vi "RGseriesSeria210216CeramicPS1.vi"() -> ()   [LabVIEW 2015]
uses:
  <vilib>/Instr/_visa.llb/VISA Configure Serial Port (Instr).vi
  <userlib>/caLab/Private/Get_PV-1D.vi
  <userlib>/caLab/Private/Put_DBL-1D_PV-1D.vi
panel:
  out "read Current":string
  out "read Voltage":string
  out "concatenated string":string
  out "ReadWait":i16
  out "WriteWait":i16
  in  "APX:PS2_T_RV":dbl
  out "APX:PS2_V_EV":dbl format="%.3f"
  out "APX:PS2_I_EV":dbl format="%.3f"
  out "Ilim_factor":dbl
  out "Vlim_factor":dbl
  out "SSE:Tsample":dbl
  in  "I lower limit":dbl
  in  "V lower limit":dbl
  in  "I upper limit":dbl=2.8
  in  "V upper limit":dbl=18.0
  out "APX:PS2_Ct":dbl
  out "APX:PS2_Rzero":dbl
  in  "Heater":u16(ring) items=["Ceramic W/Mo", "Kanthal A-1"]
  out "APX:Theater":dbl
  out "APX:PS2_R_MV":dbl format="%.2f"
  in  "REMOTE/LOCAL":bool
  out "PS2_P_MV":dbl format="%.2f"
  in  "APX:PS2_I_RV":dbl min=0.0 max=0.5 step=0.002
  in  "APX:PS2_OUT":bool
  in  "stop":bool
  out "APX:PS2_I_MV":dbl format="%.3g"
  out "APX:PS2_V_MV":dbl format="%.3g"
  in  "VISA resource name":refnum<visa-resource-name>="COM12"
  in  "APX:PS2_V_RV":dbl min=0.0 max=8.0 step=0.05
  # "COM20"
  # "#2"
  # "Sample Heater Control"
  # "COM12"
  # "V"
  # "A"
  # "Max 1.2A/0.4x0.1wire"
  # "W"
  # "ohm"
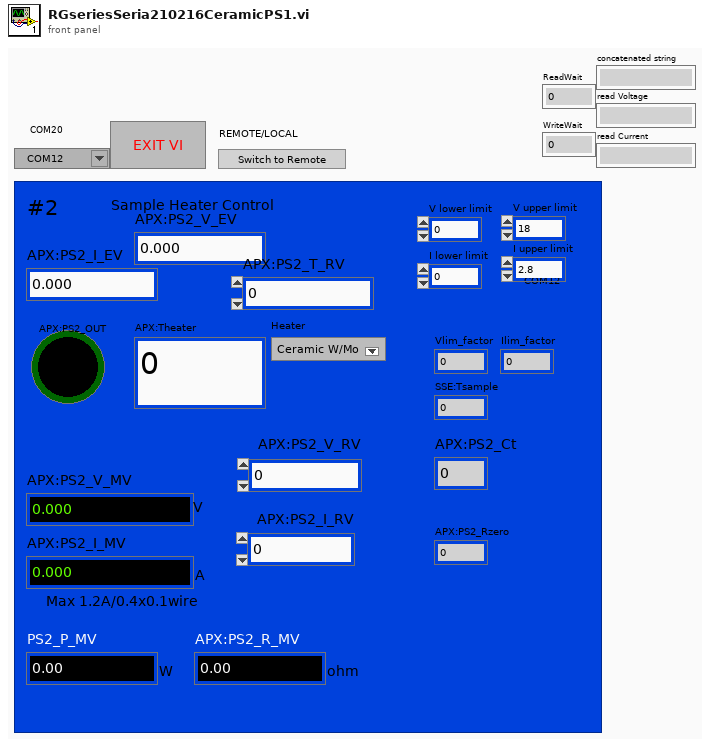
[diagram p1: front panel]
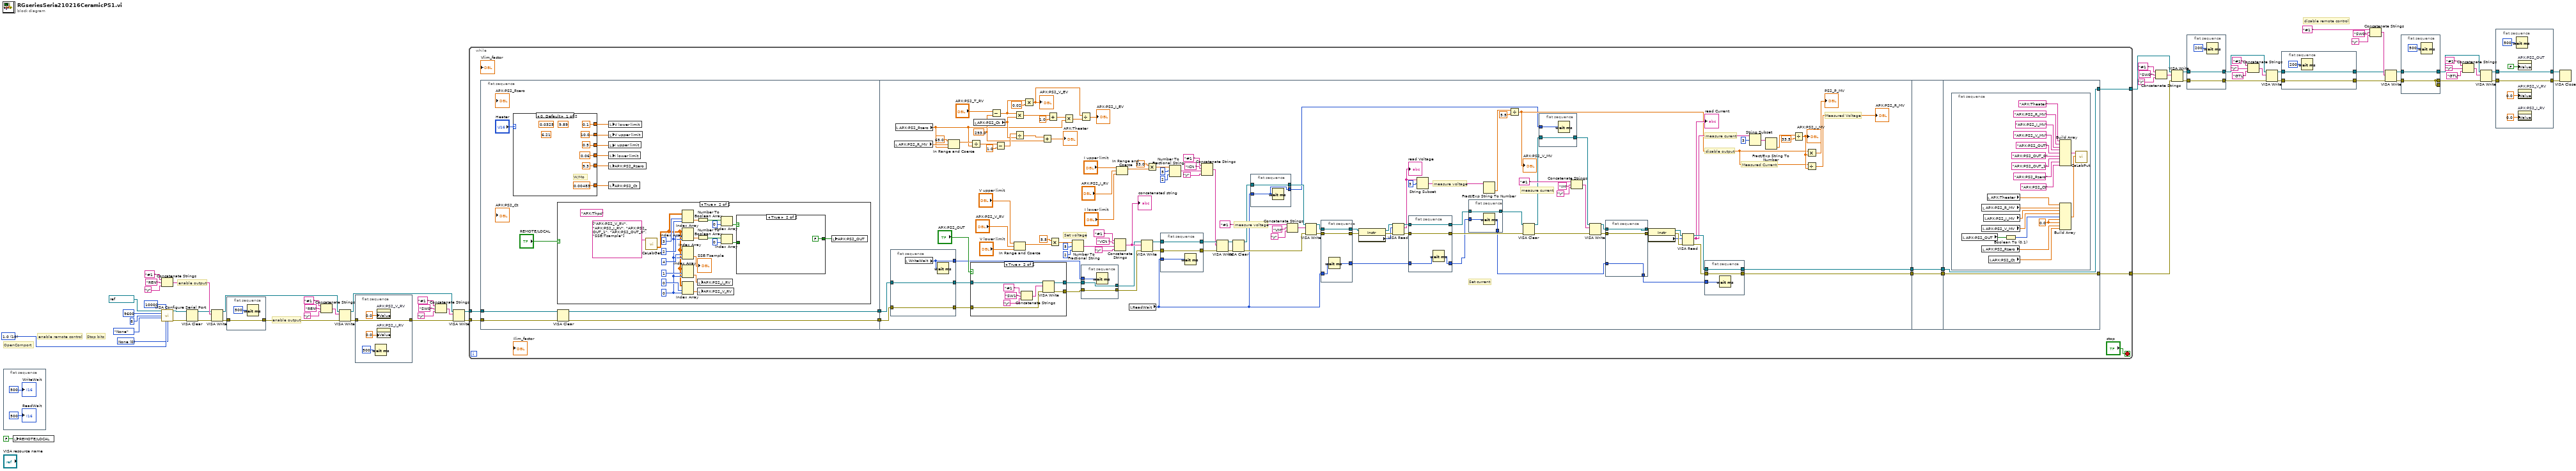
[diagram p0: block diagram]
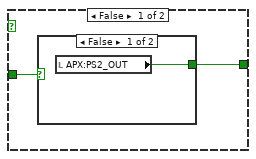
[diagram p3: hidden frame]
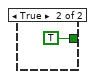
[diagram p4: hidden frame]
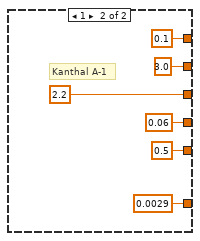
[diagram p5: hidden frame]
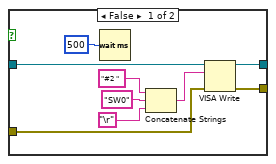
[diagram p6: hidden frame]
diagram:
  w54 = u16 0 items=["None", "XON/XOFF", "RTS/CTS", "XON/XOFF & RTS/CTS", "DTR/DSR", "XON/XOFF & DTR/DSR"] ("flow control (0:none)")
  w55 = u16 10 items=["1.0"=10, "1.5"=15, "2.0"=20] ("stop bits (10: 1 bit)")
  # "enable output"
  # "disable remote control"
  # "OpenComport"
  # "Stop bits"
  # "enable remote control"
  # "enable output"
  n1 = flat-sequence {
    frame #0 {
      "WriteWait" <- i16 500 ("WriteWait")
      "ReadWait" <- i16 500 ("ReadWait")
    }
  }
  n2 = local write "REMOTE/LOCAL"(FALSE ("REMOTE/LOCAL")) -> ()
  n3 = Concatenate Strings("#1 " ("initial string"), "REN" ("string"), "\r") -> (w53:string)
  n4 = call-poly "VISA Configure Serial Port"("VISA resource name"=refnum<visa-resource-name> "COM20", "timeout (10sec)"=u32 10000, "baud rate (9600)"=u32 9600, "data bits (8)"=u16 8, "parity (0:none)"=enum16{"None", "Odd", "Even", "Mark", "Space"}."None", "stop bits (10: 1 bit)"=w55, "flow control (0:none)"=w54) -> ("VISA resource name out"=w4:refnum<visa-resource-name>, "error out"=w3:errorcluster)  [unwired: 7 in]
  n5 = VISA Clear(VISA resource name=w4, error in (no error)=w3) -> (VISA resource name out=w1:refnum<visa-resource-name>, error out=w2:errorcluster)
  n6 = VISA Write(VISA resource name=w1, write buffer=w53, error in (no error)=w2) -> (VISA resource name out=w27:refnum<visa-resource-name>, error out=w20:errorcluster)  [unwired: 1 out]
  n7 = flat-sequence {
    tunnel: w20 -> [w70]
    tunnel: [w70] -> w21
    frame #0 {
      n8 = Wait (ms)(milliseconds to wait=u32 500) -> ()  [unwired: 1 out]
    }
  }
  n9 = Concatenate Strings("#1 " ("initial string"), "REN" ("string"), "\r") -> (w22:string)
  n10 = VISA Write(VISA resource name=w27, write buffer=w22, error in (no error)=w21) -> (VISA resource name out=w26:refnum<visa-resource-name>, error out=w19:errorcluster)  [unwired: 1 out]
  n11 = flat-sequence {
    tunnel: [w74] -> w40
    tunnel: w19 -> [w74]
    frame #0 {
      n12 = Wait (ms)(milliseconds to wait=u32 500) -> ()  [unwired: 1 out]
      n13 = property on="APX:PS2_V_RV" class="DigNum (strict)"("Value"=0.0 ("VCN_REQ")) -> ()  [unwired: 2 in, 2 out]
      n14 = property on="APX:PS2_I_RV" class="DigNum (strict)"("Value"=0.0 ("APX:RG183_I_RV")) -> ()  [unwired: 2 in, 2 out]
    }
  }
  n15 = Concatenate Strings("#1 " ("format string"), "SW0" ("initial string"), "\r" ("input 1")) -> (w52:string)
  n16 = VISA Write(VISA resource name=w26, write buffer=w52, error in (no error)=w40) -> (VISA resource name out=w42:refnum<visa-resource-name>, error out=w41:errorcluster)  [unwired: 1 out]
  n17 = while {
    tunnel: w42 -> [w84]
    tunnel: w41 -> [w85]
    tunnel: [w81] -> w39
    tunnel: [w80] -> w38
    stop <- "stop" stop-if-true
    n18 = flat-sequence {
      tunnel: w84 -> [w89]
      tunnel: w85 -> [w87]
      tunnel: [w86] -> w78
      tunnel: [w88] -> w77
      tunnel: [w198] -> w83
      tunnel: [w197] -> w82
      tunnel: w78 -> [w158]
      tunnel: w77 -> [w159]
      tunnel: w83 -> [w302]
      tunnel: w82 -> [w301]
      tunnel: [w301] -> w76
      tunnel: [w302] -> w75
      tunnel: [w304] -> w80
      tunnel: [w303] -> w81
      tunnel: w76 -> [w304]
      tunnel: w75 -> [w303]
      frame #0 {
        n19 = case shown="0, Default" "Heater" {
          tunnel: [0.00483 ("APX:PS2_Ct") 0.0029 ("APX:PS2_Ct")] -> w94
          tunnel: [9.3 ("APX:PS2_Rzero") 0.5 ("APX:PS2_Rzero")] -> w95
          tunnel: [0.5 2.2] -> w96
          tunnel: [10.0 3.0] -> w97
          tunnel: [0.1 0.1] -> w91
          tunnel: [0.06 0.06] -> w90
          frame 0, Default {
            (unwired) 9.89 ("APX:PS2_Rzero")
            (unwired) 0.0325 ("APX:PS2_Ct")
            (unwired) 6.21 ("APX:PS2_Rzero")
            # "W/Mo"
          }
          frame 1 {
            # "Kanthal A-1"
          }
        }
        n20 = case shown="True" "REMOTE/LOCAL" {
          frame False {
          }
          frame True {
            w100 = 0 ("disabled index (col)")
            (unwired) "APX:Thpc"
            n21 = call-poly "CaLabGet.vi"("PV Names"=string[] ["APX:PS2_V_RV", "APX:PS2_I_RV", "APX:PS2_OUT_1", "APX:PS2_OUT_0", "SSE:Tsample"]) -> ("Value Array (number)"=w99:dbl[][])  [unwired: 8 in, 6 out]
            n22 = Index Array(array=w99, index (row)=3 ("disabled index (row)"), index (col)=w100) -> (element=w107:dbl)
            n23 = Index Array(array=w99, index (row)=2, index (col)=w100) -> (element=w113:dbl)
            n24 = Index Array(array=w99, index (row)=4, index (col)=w100) -> (element=→"SSE:Tsample":dbl)
            n25 = Index Array(array=w99, index (row)=1, index (col)=w100) -> (element=w102:dbl)
            n26 = Index Array(array=w99, index (row)=0, index (col)=w100) -> (element=w103:dbl)
            n27 = Number To Boolean Array(number=w107) -> (Boolean array=w109:bool[])
            n28 = Number To Boolean Array(number=w113) -> (Boolean array=w112:bool[])
            n29 = local write "APX:PS2_I_RV"(w102) -> ()
            n30 = local write "APX:PS2_V_RV"(w103) -> ()
            n31 = Index Array(array=w109, index=0) -> (element=w106:bool)
            n32 = Index Array(array=w112, index=0) -> (element=w105:bool)
            n33 = case shown="True" w106 {
              tunnel: w105 -> [w119 _]
              tunnel: [w118 FALSE] -> w104
              frame False {
                n34 = case shown="False" w119 {
                  tunnel: [w120 TRUE] -> w118
                  frame False {
                    n35 = local read "APX:PS2_OUT"() -> (w120:bool)
                  }
                  frame True {
                  }
                }
              }
              frame True {
              }
            }
            n36 = local write "APX:PS2_OUT"(w104) -> ()
          }
        }
        n37 = VISA Clear(VISA resource name=w89, error in (no error)=w87) -> (VISA resource name out=w88:refnum<visa-resource-name>, error out=w86:errorcluster)
        n38 = local write "V lower limit"(w91) -> ()
        n39 = local write "V upper limit"(w97) -> ()
        n40 = local write "I upper limit"(w96) -> ()
        n41 = local write "I lower limit"(w90) -> ()
        n42 = local write "APX:PS2_Rzero"(w95) -> ()
        n43 = local write "APX:PS2_Ct"(w94) -> ()
      }
      frame #1 {
        w172 = 293.0 ("y")
        # "measure current"
        # "measure voltage"
        # "measure voltage"
        # "measure curent"
        # "Measured Voltage"
        # "Measured Current"
        # "Set current"
        # "Set voltage"
        # "disable output"
        n44 = flat-sequence {
          tunnel: w159 -> [w260]
          tunnel: w158 -> [w259]
          tunnel: [w260] -> w156
          tunnel: [w259] -> w157
          tunnel: [w258] -> w155
          frame #0 {
            n45 = local read "WriteWait"() -> (w258:i16)
            n46 = Wait (ms)(milliseconds to wait=w258) -> ()  [unwired: 1 out]
          }
        }
        n47 = local read "APX:PS2_R_MV"() -> (w185:dbl)
        n48 = local read "APX:PS2_Rzero"() -> (w167:dbl)
        n49 = In Range and Coerce(upper limit=65.0, x=w185, lower limit=w167) -> (coerced(x)=w183:dbl)  [unwired: 1 out]
        n50 = Divide(x=w183, y=w167) -> (x/y=w182:dbl)
        n51 = case shown="True" "APX:PS2_OUT" {
          tunnel: w156 -> [w270 w279]
          tunnel: w157 -> [w269 w278]
          tunnel: [w268 w277] -> w196
          tunnel: [w267 w276] -> w195
          frame False {
            n52 = Wait (ms)(milliseconds to wait=u32 500) -> ()  [unwired: 1 out]
            n53 = Concatenate Strings("#2 " ("format string"), "SW0" ("initial string"), "\r" ("input 1")) -> (w272:string)
            n54 = VISA Write(VISA resource name=w270, write buffer=w272, error in (no error)=w269) -> (VISA resource name out=w267:refnum<visa-resource-name>, error out=w268:errorcluster)  [unwired: 1 out]
          }
          frame True {
            n55 = Concatenate Strings("#1 " ("format string"), "SW1" ("initial string"), "\r" ("input 1")) -> (w280:string)
            n56 = VISA Write(VISA resource name=w279, write buffer=w280, error in (no error)=w278) -> (VISA resource name out=w276:refnum<visa-resource-name>, error out=w277:errorcluster)  [unwired: 1 out]
          }
        }
        n57 = local read "APX:PS2_Ct"() -> (w171:dbl)
        n58 = Subtract(x="APX:PS2_T_RV", y=w172) -> (x-y=w166:dbl)
        n59 = Subtract(x=w182, y=1.0) -> (x-y=w180:dbl)
        n60 = Multiply(x=w166, y=w171) -> (x*y=w170:dbl)
        n61 = Divide(x=w180, y=w171) -> (x/y=w179:dbl)
        n62 = In Range and Coerce(upper limit="V upper limit", x="APX:PS2_V_RV", lower limit="V lower limit") -> (coerced(x)=w193:dbl)  [unwired: 1 out]
        n63 = Multiply(x=w166, y=0.02) -> (x*y=w162:dbl)
        "APX:PS2_V_EV" <- w162
        n64 = Add(x=w179, y=w172) -> (x+y=→"APX:Theater":dbl)
        n65 = Add(x=w170, y=1.0) -> (x+y=w168:dbl)
        n66 = Multiply(x=5.5, y=w193) -> (x*y=w251:dbl)
        n67 = Multiply(x=w168, y=w167) -> (x*y=w163:dbl)
        n68 = Number To Fractional String(number=w251, width (-)=i16 5, precision (6)=i16 2) -> (F-format string=w252:string)  [unwired: 1 in]
        n69 = Divide(x=w162, y=w163) -> (x/y=→"APX:PS2_I_EV":dbl)
        n70 = flat-sequence {
          tunnel: w195 -> [w299]
          tunnel: w196 -> [w300]
          tunnel: [w300] -> w199
          tunnel: [w299] -> w200
          tunnel: w155 -> [w298]
          frame #0 {
            n71 = Wait (ms)(milliseconds to wait=w298) -> ()  [unwired: 1 out]
          }
        }
        n72 = Concatenate Strings("#1 " ("format string"), "VCN " ("initial string"), w252, "\r") -> (w203:string)
        "concatenated string" <- w203
        n73 = In Range and Coerce(upper limit="I upper limit", x="APX:PS2_I_RV", lower limit="I lower limit") -> (coerced(x)=w191:dbl)  [unwired: 1 out]
        n74 = local read "ReadWait"() -> (w141:i16)
        n75 = VISA Write(VISA resource name=w200, write buffer=w203, error in (no error)=w199) -> (VISA resource name out=w161:refnum<visa-resource-name>, error out=w160:errorcluster)  [unwired: 1 out]
        n76 = Multiply(x=33.0, y=w191) -> (x*y=w241:dbl)
        n77 = flat-sequence {
          tunnel: w161 -> [w266]
          tunnel: w160 -> [w265]
          tunnel: [w266] -> w146
          tunnel: [w265] -> w145
          tunnel: w141 -> [w264]
          frame #0 {
            n78 = Wait (ms)(milliseconds to wait=w264) -> ()  [unwired: 1 out]
          }
        }
        n79 = Number To Fractional String(number=w241, width (-)=i16 5, precision (6)=i16 2) -> (F-format string=w244:string)  [unwired: 1 in]
        n80 = Concatenate Strings("#1 " ("initial string"), "ICN " ("initial string"), w244, "\r") -> (w144:string)
        n81 = VISA Write(VISA resource name=w146, write buffer=w144, error in (no error)=w145) -> (VISA resource name out=w142:refnum<visa-resource-name>, error out=w143:errorcluster)  [unwired: 1 out]
        n82 = VISA Clear(VISA resource name=w142, error in (no error)=w143) -> (VISA resource name out=w151:refnum<visa-resource-name>, error out=w154:errorcluster)
        n83 = flat-sequence {
          tunnel: w141 -> [w256]
          tunnel: w151 -> [w257]
          tunnel: [w257] -> w150
          tunnel: [w256] -> w147
          frame #0 {
            n84 = Wait (ms)(milliseconds to wait=w256) -> ()  [unwired: 1 out]
          }
        }
        n85 = Concatenate Strings("#1 " ("format string"), "VM" ("initial string"), "\r" ("input 1")) -> (w228:string)
        n86 = VISA Write(VISA resource name=w150, write buffer=w228, error in (no error)=w154) -> (VISA resource name out=w217:refnum<visa-resource-name>, error out=w215:errorcluster)  [unwired: 1 out]
        n87 = flat-sequence {
          tunnel: w217 -> [w297]
          tunnel: [w297] -> w216
          tunnel: w215 -> [w296]
          tunnel: [w296] -> w214
          tunnel: w141 -> [w295]
          tunnel: [w294] -> w140
          frame #0 {
            n88 = Wait (ms)(milliseconds to wait=w295) -> (millisecond timer value=w294:u32)
          }
        }
        n89 = property class="Instr"(reference=w216, error in=w214) -> (reference out=w223:refnum<visa-resource-name>, error out=w222:errorcluster, "Serial Settings:Number of Bytes at Serial Port"=w221:u32)
        n90 = VISA Read(VISA resource name=w223, byte count=w221, error in (no error)=w222) -> (VISA resource name out=w209:refnum<visa-resource-name>, read buffer=w204:string, error out=w208:errorcluster)  [unwired: 1 out]
        "read Voltage" <- w204
        n91 = flat-sequence {
          tunnel: w209 -> [w290]
          tunnel: w208 -> [w289]
          tunnel: [w290] -> w139
          tunnel: [w287] -> w137
          tunnel: w140 -> [w288]
          tunnel: [w289] -> w138
          frame #0 {
            n92 = Wait (ms)(milliseconds to wait=w288) -> (millisecond timer value=w287:u32)
          }
        }
        n93 = String Subset(string=w204, offset (0)=3) -> (substring=w202:string)  [unwired: 1 in]
        n94 = flat-sequence {
          tunnel: w139 -> [w263]
          tunnel: [w263] -> w153
          tunnel: w137 -> [w262]
          tunnel: [w261] -> w136
          frame #0 {
            n95 = Wait (ms)(milliseconds to wait=w262) -> (millisecond timer value=w261:u32)
          }
        }
        n96 = Fract/Exp String To Number(string=w202) -> (number=w237:dbl)  [unwired: 3 in, 1 out]
        n97 = Divide(x=w237, y=5.5 ("x")) -> (x/y=w188:dbl)
        "APX:PS2_V_MV" <- w188
        n98 = VISA Clear(VISA resource name=w153, error in (no error)=w138) -> (VISA resource name out=w149:refnum<visa-resource-name>, error out=w152:errorcluster)
        n99 = flat-sequence {
          tunnel: w147 -> [w255]
          tunnel: w149 -> [w254]
          tunnel: [w254] -> w148
          frame #0 {
            n100 = Wait (ms)(milliseconds to wait=w255) -> ()  [unwired: 1 out]
          }
        }
        n101 = Concatenate Strings("#1 " ("format string"), "IM" ("initial string"), "\r" ("input 1")) -> (w225:string)
        n102 = VISA Write(VISA resource name=w148, write buffer=w225, error in (no error)=w152) -> (VISA resource name out=w213:refnum<visa-resource-name>, error out=w212:errorcluster)  [unwired: 1 out]
        n103 = flat-sequence {
          tunnel: w213 -> [w293]
          tunnel: w212 -> [w292]
          tunnel: [w293] -> w211
          tunnel: [w292] -> w210
          tunnel: w136 -> [w291]
          tunnel: [w291] -> w135
          frame #0 {
          }
        }
        n104 = property class="Instr"(reference=w211, error in=w210) -> (reference out=w220:refnum<visa-resource-name>, error out=w219:errorcluster, "Serial Settings:Number of Bytes at Serial Port"=w218:u32)
        n105 = VISA Read(VISA resource name=w220, byte count=w218, error in (no error)=w219) -> (VISA resource name out=w207:refnum<visa-resource-name>, read buffer=w205:string, error out=w206:errorcluster)  [unwired: 1 out]
        "read Current" <- w205
        n106 = flat-sequence {
          tunnel: w207 -> [w286]
          tunnel: w206 -> [w285]
          tunnel: [w286] -> w198
          tunnel: [w285] -> w197
          tunnel: w135 -> [w284]
          frame #0 {
            n107 = Wait (ms)(milliseconds to wait=w284) -> ()  [unwired: 1 out]
          }
        }
        n108 = String Subset(string=w205, offset (0)=3) -> (substring=w201:string)  [unwired: 1 in]
        n109 = Fract/Exp String To Number(string=w201) -> (number=w234:dbl)  [unwired: 3 in, 1 out]
        n110 = Divide(x=w234, y=33.5 ("x")) -> (x/y=w189:dbl)
        "APX:PS2_I_MV" <- w189
        n111 = Multiply(x=w188, y=w189) -> (x*y=→"PS2_P_MV":dbl)
        n112 = Divide(x=w188, y=w189) -> (x/y=→"APX:PS2_R_MV":dbl)
      }
      frame #2 {
      }
      frame #3 {
        n113 = flat-sequence {
          frame #0 {
            w309 = 0.0 ("element")
            n114 = local read "APX:PS2_OUT"() -> (w313:bool)
            n115 = local read "APX:PS2_R_MV"() -> (w318:dbl)
            n116 = local read "APX:PS2_V_MV"() -> (w316:dbl)
            n117 = local read "APX:PS2_Rzero"() -> (w305:dbl)
            n118 = local read "APX:PS2_I_MV"() -> (w317:dbl)
            n119 = local read "APX:Theater"() -> (w319:dbl)
            n120 = local read "APX:PS2_Ct"() -> (w306:dbl)
            n121 = Boolean To (0,1)(Boolean=w313) -> (0, 1=w312:i16)
            n122 = Build Array("APX:Theater", "APX:PS2_R_MV", "APX:PS2_I_MV", "APX:PS2_V_MV", "APX:PS2_OUT", "APX:PS2_OUT_0", "APX:PS2_OUT_1", "APX:PS2_Rzero", "APX:PS2_Ct") -> (w324:string[])
            n123 = Build Array(w319, w318, w317, w316, w312, w309, w309, w305, w306) -> (w315:dbl[])
            n124 = call-poly <userlib>:"CaLabPut.vi"("Values"=w315, "PV Names"=w324) -> ()  [unwired: 6 in, 4 out]
          }
        }
      }
    }
  }
  n125 = Concatenate Strings("#1 " ("format string"), "SW0" ("initial string"), "\r" ("input 1")) -> (w46:string)
  n126 = VISA Write(VISA resource name=w39, write buffer=w46, error in (no error)=w38) -> (VISA resource name out=w16:refnum<visa-resource-name>, error out=w14:errorcluster)  [unwired: 1 out]
  n127 = flat-sequence {
    tunnel: w16 -> [w325]
    tunnel: w14 -> [w327]
    tunnel: [w325] -> w15
    tunnel: [w327] -> w13
    frame #0 {
      n128 = Wait (ms)(milliseconds to wait=u32 200) -> ()  [unwired: 1 out]
    }
  }
  n129 = Concatenate Strings("#1" ("initial string"), "\r", "GTL" ("input 1")) -> (w51:string)
  n130 = VISA Write(VISA resource name=w15, write buffer=w51, error in (no error)=w13) -> (VISA resource name out=w8:refnum<visa-resource-name>, error out=w7:errorcluster)  [unwired: 1 out]
  n131 = flat-sequence {
    tunnel: w8 -> [w330]
    tunnel: w7 -> [w329]
    tunnel: [w330] -> w6
    tunnel: [w329] -> w5
    frame #0 {
      n132 = Wait (ms)(milliseconds to wait=u32 200) -> ()  [unwired: 1 out]
    }
  }
  n133 = Concatenate Strings("#1 " ("format string"), "SW0" ("initial string"), "\r" ("input 1")) -> (w33:string)
  n134 = VISA Write(VISA resource name=w6, write buffer=w33, error in (no error)=w5) -> (VISA resource name out=w12:refnum<visa-resource-name>, error out=w10:errorcluster)  [unwired: 1 out]
  n135 = flat-sequence {
    tunnel: w12 -> [w333]
    tunnel: w10 -> [w331]
    tunnel: [w333] -> w11
    tunnel: [w331] -> _
    tunnel: [w331] -> w9
    frame #0 {
      n136 = Wait (ms)(milliseconds to wait=u32 500) -> ()  [unwired: 1 out]
    }
  }
  n137 = Concatenate Strings("#1" ("initial string"), "\r", "GTL" ("input 1")) -> (w34:string)
  n138 = VISA Write(VISA resource name=w11, write buffer=w34, error in (no error)=w9) -> (VISA resource name out=w29:refnum<visa-resource-name>, error out=w28:errorcluster)  [unwired: 1 out]
  n139 = flat-sequence {
    tunnel: w29 -> [w338]
    tunnel: w28 -> [w337]
    tunnel: [w338] -> w48
    tunnel: [w337] -> w47
    frame #0 {
      n140 = Wait (ms)(milliseconds to wait=u32 500) -> ()  [unwired: 1 out]
      n141 = property on="APX:PS2_OUT" class="Bool (strict)"("Value"=FALSE ("Output")) -> ()  [unwired: 2 in, 2 out]
      n142 = property on="APX:PS2_V_RV" class="DigNum (strict)"("Value"=0.0 ("VCN_REQ")) -> ()  [unwired: 2 in, 2 out]
      n143 = property on="APX:PS2_I_RV" class="DigNum (strict)"("Value"=0.0 ("APX:RG183_I_RV")) -> ()  [unwired: 2 in, 2 out]
    }
  }
  n144 = VISA Close(VISA resource name=w48, error in (no error)=w47) -> ()  [unwired: 1 out]
